vi "GeneratorCpkReport.vi"(4 "结束行in":string, 6 "起始行in":string, 8 "error in (no error)":errorcluster caption="错误输入（无错误）", 10 "测试数据in":string[][](array[string]), 11 "路径in":path) -> (0 "error out":errorcluster caption="错误输出")   [LabVIEW 2020]
uses:
  <vilib>/Utility/NIReport.llb/Report Type.ctl
  <vilib>/addons/_office/_exclsub.llb/font.ctl
  <vilib>/Utility/NIReport.llb/Append Text Table to Report (wrap).vi
  <vilib>/Utility/NIReport.llb/NI_report.lvclass
  <vilib>/Utility/NIReport.llb/NI_ReportGenerationCore.lvlib
  <vilib>/addons/_office/NI_ReportGenerationToolkit.lvlib
  <vilib>/Utility/NIReport.llb/Excel/NI_Excel.lvclass
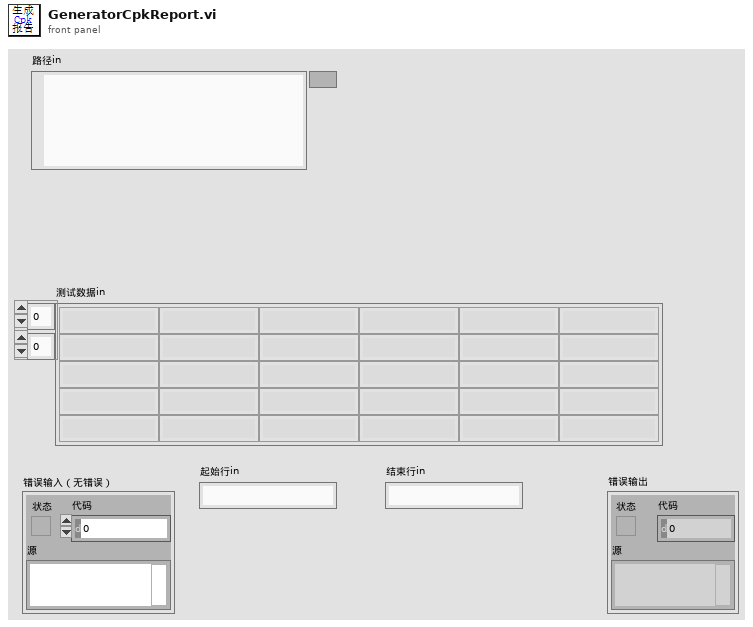
[diagram p1: front panel]
types:
  T1 = cluster{"on/off":bool, "weight":i32, "color":u32}
  T2 = cluster{"position (excel)":cluster{"row":i32, "column":i32}, "name (excel)":string, "bookmark (word)":string}
  T3 = typedef "NI_ReportGenerationToolkit.lvlib/font.ctl" = cluster{"font name":string, "font size":dbl, "bold":u16, "italic":u16, "underline":u16, "strike through":u16, "font color":u32}
  T4 = enum16{"maximized", "minimized", "normal", "no change"}
  T5 = typedef "NI_ReportGenerationCore.lvlib/Report Type.ctl" = enum16{"HTML", "Word", "Excel"}
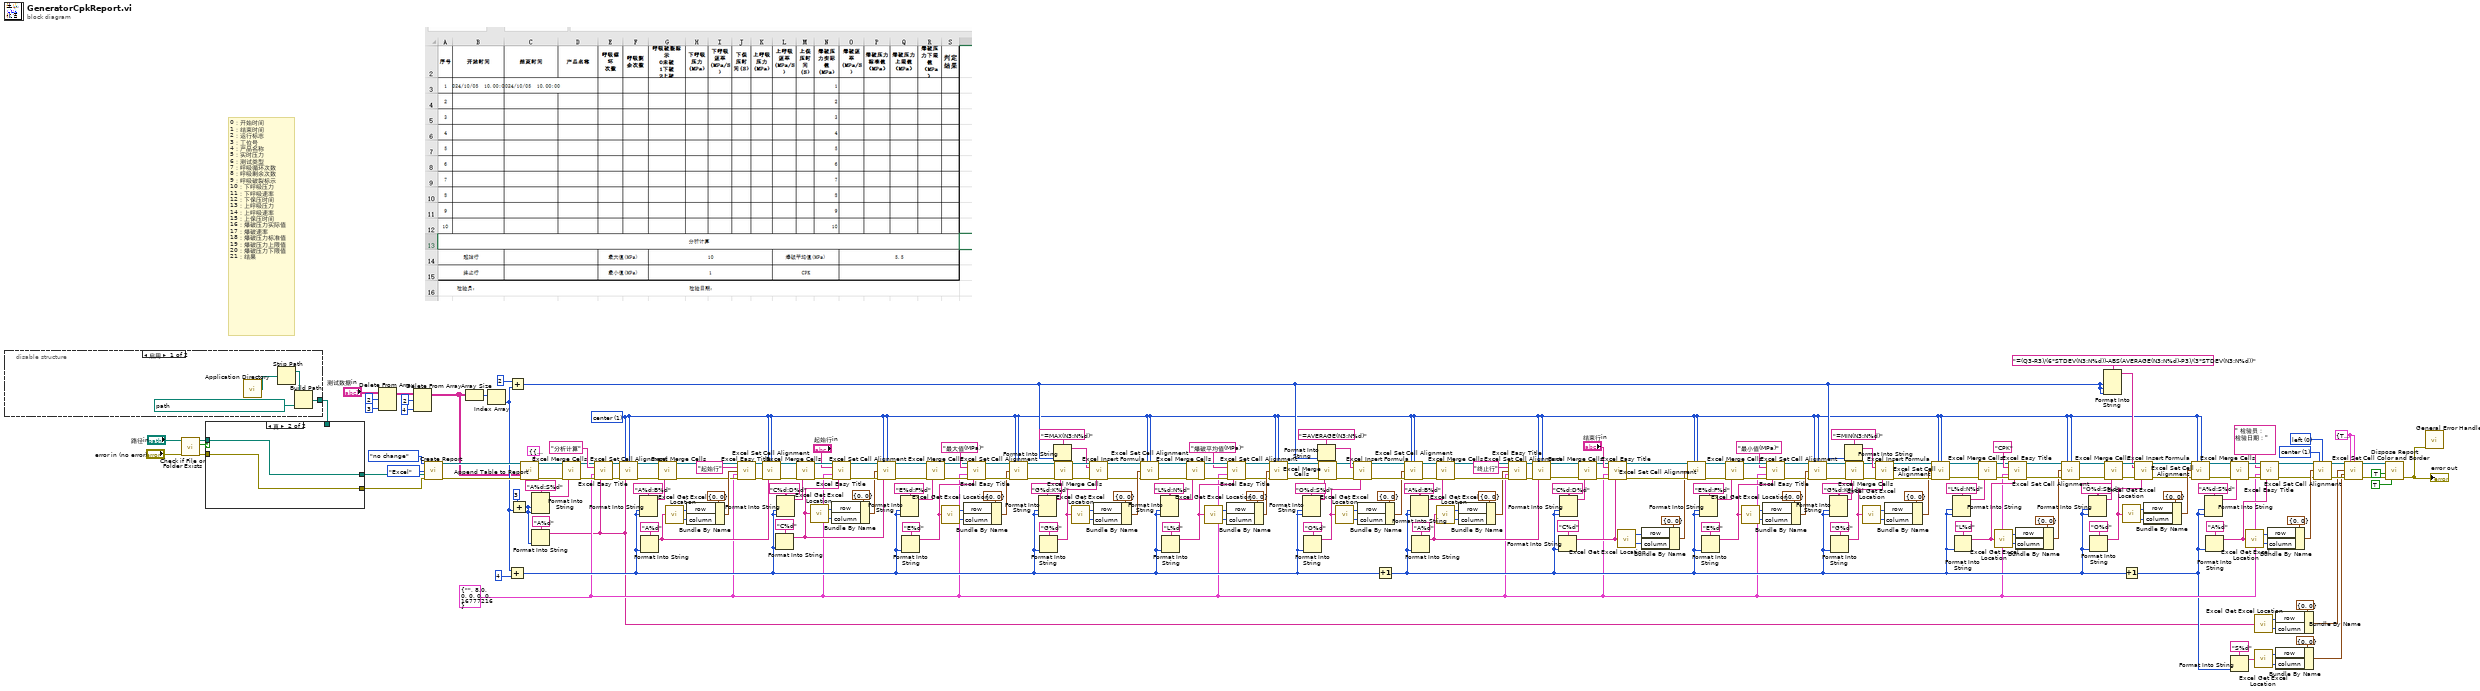
[diagram p0: block diagram]
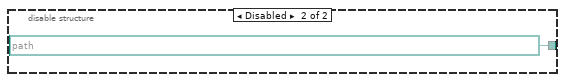
[diagram p2: hidden frame]
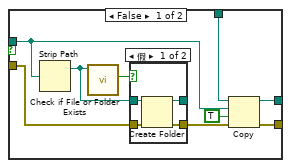
[diagram p3: hidden frame]
diagram:
  w13 = T1 {"on/off"=TRUE, "weight"=2, "color"=0} ("inside border")
  w27 = 0 items=["left", "center", "right"] ("horizontal alignment (left)")
  w28 = 1 items=["top", "center", "bottom"] ("vertical alignment (top)")
  w29 = 1 items=["top", "center", "bottom"] ("vertical alignment (top)")
  w25 = T3 {"font name"="", "font size"=8.0, "bold"=0, "italic"=0, "underline"=0, "strike through"=0, "font color"=16777216} ("font")
  # "0：开始时间\n1：结束时间\n2：运行标志\n3：工位号\n4：产品名称\n5：实时压力\n6：测试类型\n7：呼吸循环次数\n8：呼吸剩余次数\n9：呼吸破裂标示\n10：下呼吸压力\n11：下呼吸速率\n12：下保压时间\n13：上呼吸压力\n14：上呼吸速率\n15：上保压时间\n16：爆破压力实际值\n17：爆破速率\n18：爆破压力标准值\n19：爆破压力上限值\n20：爆破压力下限值\n21：结果"
  n1 = disable-structure shown="启用" {
    disable-tunnel: [w265 path "D:/KebodaWork/深圳何军生/呼吸测试台/SourceCode/Config/呼吸爆破测试CPK最新模板.xlsx" ("appended path")] -> w259
    frame Enabled {
      n2 = call <vilib>:"Application Directory.vi"() -> ("Application Directory"=w264:path)
      n3 = Strip Path(path=w264) -> (stripped path=w263:path)  [unwired: 1 out]
      n4 = Build Path(base path=w263, name or relative path=path "Config/呼吸爆破测试CPK最新模板.xlsx" ("名称或相对路径")) -> (appended path=w265:path)
    }
    frame Disabled {
    }
  }
  n5 = call <vilib>:"Check if File or Folder Exists.vi"("error in (no error)"="error in (no error)", "path"="路径in") -> ("error out"=w261:errorcluster, "file or folder exists?"=w262:bool, "dup path"=w260:path)  [unwired: 7 in]
  n6 = case shown="真" w262 {
    tunnel: w261 -> [w276 w284]
    tunnel: w260 -> [w268 w283]
    tunnel: [w273 w284] -> w253
    tunnel: w259 -> [w270 _]
    tunnel: [w271 w283] -> w254
    frame False {
      n7 = Strip Path(path=w268) -> (stripped path=w275:path)  [unwired: 1 out]
      n8 = call <vilib>:"Check if File or Folder Exists.vi"("path"=w275) -> ("file or folder exists?"=w274:bool)  [unwired: 8 in, 2 out]
      n9 = case shown="假" w274 {
        tunnel: w276 -> [w280 w282]
        tunnel: [w279 w282] -> w269
        tunnel: w275 -> [w278 w281]
        tunnel: [w277 w281] -> _
        frame False {
          n10 = Create Folder(path (use dialog)=w278, error in=w280) -> (created path=w277:path, error out=w279:errorcluster)  [unwired: 1 in, 1 out]
        }
        frame True {
        }
      }
      n11 = Copy(8:w269, 9:TRUE ("覆盖(F)"), 10:w268, 11:w270) -> (0:w273:errorcluster, 3:w271:path)  [unwired: 1 in, 1 out]
    }
    frame True {
    }
  }
  n12 = Delete From Array(array="测试数据in", length=2 ("禁用的索引 (列)"), index (col)=3 ("禁用的索引 (列)")) -> (array with subset deleted=w23:string[][])  [unwired: 1 in, 1 out]
  n13 = Delete From Array(array=w23, length=2 ("禁用的索引 (列)"), index (col)=4 ("禁用的索引 (列)")) -> (array with subset deleted=w20:string[][])  [unwired: 1 in, 1 out]
  n14 = call <vilib>:"Create Report.vi"("window state (normal)"=T4."no change", "report type"=Report_Type."Excel", "template (empty)"=w254, "error in (no error)"=w253) -> ("report out"=w241:refnum<class "NI_report.lvclass">, "error out"=w240:errorcluster)  [unwired: 10 in]
  n15 = Array Size(array=w20) -> (size(s)=w236:i32[])
  n16 = Index Array(array=w236) -> (element=w170:i32)  [unwired: 1 in]
  n17 = Add(x=w170, y=4) -> (x+y=w26:i32)
  n18 = Add(x=2, y=w170) -> (x+y=w46:i32)
  n19 = Add(x=3 ("y"), y=w170) -> (x+y=w226:i32)
  n20 = call-poly <vilib>:"Append Table to Report.vi"("report in"=w241, "MS Office parameters"=T2 {"position (excel)"={"row"=2, "column"=0}, "name (excel)"="", "bookmark (word)"=""}, "text data"=w20, "error in (no error)"=w240) -> ("report out"=w231:refnum<class "NI_report.lvclass">, "error out"=w233:errorcluster)  [unwired: 8 in, 2 out]
  n21 = Format Into String(format string="A%d:S%d" ("格式字符串"), w226, w226) -> (resulting string=w228:string)  [unwired: 2 in, 1 out]
  n22 = Format Into String(format string="A%d" ("格式字符串"), w226) -> (resulting string=w1:string)  [unwired: 2 in, 1 out]
  n23 = call <vilib>:"Excel Merge Cells.vi"("report in"=w231, "error in (no error)"=w233, "name (\"\")"=w228) -> ("report out"=w230:refnum<class "NI_report.lvclass">, "error out"=w232:errorcluster)  [unwired: 11 in]
  n24 = call <vilib>:"Excel Easy Title.vi"("report in"=w230, "title"="分析计算", "font"=w25, "error in (no error)"=w232, "name (\"\")"=w1) -> ("report out"=w225:refnum<class "NI_report.lvclass">, "error out"=w224:errorcluster)  [unwired: 8 in, 1 out]
  n25 = call <vilib>:"Excel Set Cell Alignment.vi"("report in"=w225, "vertical alignment (top)"=w29, "horizontal alignment (left)"=w29, "error in (no error)"=w224, "name (\"\")"=w1) -> ("report out"=w221:refnum<class "NI_report.lvclass">, "error out"=w219:errorcluster)  [unwired: 9 in]
  n26 = Format Into String(format string="A%d:B%d" ("格式字符串"), w26, w26) -> (resulting string=w223:string)  [unwired: 2 in, 1 out]
  n27 = Format Into String(format string="A%d" ("格式字符串"), w26) -> (resulting string=w200:string)  [unwired: 2 in, 1 out]
  n28 = call <vilib>:"Excel Merge Cells.vi"("report in"=w221, "error in (no error)"=w219, "name (\"\")"=w223) -> ("report out"=w220:refnum<class "NI_report.lvclass">, "error out"=w218:errorcluster)  [unwired: 11 in]
  n29 = call <vilib>:"Excel Get Excel Location.vi"("cell's name"=w200) -> ("row"=w248:i32, "column"=w247:i32)
  n30 = Bundle By Name(cluster=cluster{"row":i32, "column":i32} {"row"=0, "column"=0} ("start (0, 0)"), "row"=w248, "column"=w247) -> (w246:cluster{"row":i32, "column":i32})
  n31 = call <vilib>:"Excel Easy Title.vi"("report in"=w220, "title"="起始行", "start (0, 0)"=w246, "font"=w25, "error in (no error)"=w218) -> ("report out"=w214:refnum<class "NI_report.lvclass">, "error out"=w215:errorcluster)  [unwired: 8 in, 1 out]
  n32 = call <vilib>:"Excel Set Cell Alignment.vi"("report in"=w214, "vertical alignment (top)"=w29, "horizontal alignment (left)"=w29, "error in (no error)"=w215, "name (\"\")"=w200) -> ("report out"=w201:refnum<class "NI_report.lvclass">, "error out"=w202:errorcluster)  [unwired: 9 in]
  n33 = Format Into String(format string="C%d" ("格式字符串"), w26) -> (resulting string=w165:string)  [unwired: 2 in, 1 out]
  n34 = Format Into String(format string="C%d:D%d" ("格式字符串"), w26, w26) -> (resulting string=w208:string)  [unwired: 2 in, 1 out]
  n35 = call <vilib>:"Excel Merge Cells.vi"("report in"=w201, "error in (no error)"=w202, "name (\"\")"=w208) -> ("report out"=w210:refnum<class "NI_report.lvclass">, "error out"=w211:errorcluster)  [unwired: 11 in]
  n36 = call <vilib>:"Excel Get Excel Location.vi"("cell's name"=w165) -> ("row"=w205:i32, "column"=w206:i32)
  n37 = Bundle By Name(cluster=cluster{"row":i32, "column":i32} {"row"=0, "column"=0} ("start (0, 0)"), "row"=w205, "column"=w206) -> (w166:cluster{"row":i32, "column":i32})
  n38 = call <vilib>:"Excel Easy Title.vi"("report in"=w210, "title"="起始行in", "font"=w25, "error in (no error)"=w211, "name (\"\")"=w165) -> ("report out"=w213:refnum<class "NI_report.lvclass">, "error out"=w212:errorcluster)  [unwired: 8 in, 1 out]
  n39 = call <vilib>:"Excel Set Cell Alignment.vi"("report in"=w213, "vertical alignment (top)"=w29, "horizontal alignment (left)"=w29, "start (-1, -1)"=w166, "error in (no error)"=w212, "name (\"\")"=w165) -> ("report out"=w187:refnum<class "NI_report.lvclass">, "error out"=w188:errorcluster)  [unwired: 8 in]
  n40 = Format Into String(format string="E%d:F%d" ("格式字符串"), w26, w26) -> (resulting string=w194:string)  [unwired: 2 in, 1 out]
  n41 = Format Into String(format string="E%d" ("格式字符串"), w26) -> (resulting string=w167:string)  [unwired: 2 in, 1 out]
  n42 = call <vilib>:"Excel Merge Cells.vi"("report in"=w187, "error in (no error)"=w188, "name (\"\")"=w194) -> ("report out"=w195:refnum<class "NI_report.lvclass">, "error out"=w196:errorcluster)  [unwired: 11 in]
  n43 = call <vilib>:"Excel Get Excel Location.vi"("cell's name"=w167) -> ("row"=w192:i32, "column"=w193:i32)
  n44 = Bundle By Name(cluster=cluster{"row":i32, "column":i32} {"row"=0, "column"=0} ("start (0, 0)"), "row"=w192, "column"=w193) -> (w168:cluster{"row":i32, "column":i32})
  n45 = call <vilib>:"Excel Easy Title.vi"("report in"=w195, "title"="最大值(MPa)", "font"=w25, "error in (no error)"=w196, "name (\"\")"=w167) -> ("report out"=w199:refnum<class "NI_report.lvclass">, "error out"=w198:errorcluster)  [unwired: 8 in, 1 out]
  n46 = call <vilib>:"Excel Set Cell Alignment.vi"("report in"=w199, "vertical alignment (top)"=w29, "horizontal alignment (left)"=w29, "start (-1, -1)"=w168, "error in (no error)"=w198) -> ("report out"=w171:refnum<class "NI_report.lvclass">, "error out"=w172:errorcluster)  [unwired: 9 in]
  n47 = Format Into String(format string="G%d:K%d" ("格式字符串"), w26, w26) -> (resulting string=w181:string)  [unwired: 2 in, 1 out]
  n48 = Format Into String(format string="G%d" ("格式字符串"), w26) -> (resulting string=w178:string)  [unwired: 2 in, 1 out]
  n49 = Format Into String(format string="=MAX(N3:N%d)" ("格式字符串"), w46) -> (resulting string=w173:string)  [unwired: 2 in, 1 out]
  n50 = call <vilib>:"Excel Merge Cells.vi"("report in"=w171, "error in (no error)"=w172, "name (\"\")"=w181) -> ("report out"=w175:refnum<class "NI_report.lvclass">, "error out"=w177:errorcluster)  [unwired: 11 in]
  n51 = call <vilib>:"Excel Get Excel Location.vi"("cell's name"=w178) -> ("row"=w183:i32, "column"=w182:i32)
  n52 = call <vilib>:"Excel Insert Formula.vi"("report in"=w175, "formula"=w173, "error in (no error)"=w177, "name (\"\")"=w178) -> ("report out"=w174:refnum<class "NI_report.lvclass">, "error out"=w176:errorcluster)  [unwired: 10 in]
  n53 = Bundle By Name(cluster=cluster{"row":i32, "column":i32} {"row"=0, "column"=0} ("start (0, 0)"), "row"=w183, "column"=w182) -> (w179:cluster{"row":i32, "column":i32})
  n54 = call <vilib>:"Excel Set Cell Alignment.vi"("report in"=w174, "vertical alignment (top)"=w29, "horizontal alignment (left)"=w29, "start (-1, -1)"=w179, "error in (no error)"=w176) -> ("report out"=w150:refnum<class "NI_report.lvclass">, "error out"=w151:errorcluster)  [unwired: 9 in]
  n55 = Format Into String(format string="L%d:N%d" ("格式字符串"), w26, w26) -> (resulting string=w157:string)  [unwired: 2 in, 1 out]
  n56 = Format Into String(format string="L%d" ("格式字符串"), w26) -> (resulting string=w164:string)  [unwired: 2 in, 1 out]
  n57 = call <vilib>:"Excel Merge Cells.vi"("report in"=w150, "error in (no error)"=w151, "name (\"\")"=w157) -> ("report out"=w156:refnum<class "NI_report.lvclass">, "error out"=w155:errorcluster)  [unwired: 11 in]
  n58 = call <vilib>:"Excel Get Excel Location.vi"("cell's name"=w164) -> ("row"=w159:i32, "column"=w158:i32)
  n59 = Bundle By Name(cluster=cluster{"row":i32, "column":i32} {"row"=0, "column"=0} ("start (0, 0)"), "row"=w159, "column"=w158) -> (w163:cluster{"row":i32, "column":i32})
  n60 = call <vilib>:"Excel Easy Title.vi"("report in"=w156, "title"="爆破平均值(MPa)", "font"=w25, "error in (no error)"=w155, "name (\"\")"=w164) -> ("report out"=w152:refnum<class "NI_report.lvclass">, "error out"=w153:errorcluster)  [unwired: 8 in, 1 out]
  n61 = call <vilib>:"Excel Set Cell Alignment.vi"("report in"=w152, "vertical alignment (top)"=w29, "horizontal alignment (left)"=w29, "start (-1, -1)"=w163, "error in (no error)"=w153) -> ("report out"=w134:refnum<class "NI_report.lvclass">, "error out"=w135:errorcluster)  [unwired: 9 in]
  n62 = Format Into String(format string="O%d:S%d" ("格式字符串"), w26, w26) -> (resulting string=w141:string)  [unwired: 2 in, 1 out]
  n63 = Format Into String(format string="O%d" ("格式字符串"), w26) -> (resulting string=w144:string)  [unwired: 2 in, 1 out]
  n64 = Format Into String(format string="=AVERAGE(N3:N%d)" ("格式字符串"), w46) -> (resulting string=w149:string)  [unwired: 2 in, 1 out]
  n65 = call <vilib>:"Excel Merge Cells.vi"("report in"=w134, "error in (no error)"=w135, "name (\"\")"=w141) -> ("report out"=w147:refnum<class "NI_report.lvclass">, "error out"=w145:errorcluster)  [unwired: 11 in]
  n66 = call <vilib>:"Excel Get Excel Location.vi"("cell's name"=w144) -> ("row"=w139:i32, "column"=w140:i32)
  n67 = call <vilib>:"Excel Insert Formula.vi"("report in"=w147, "formula"=w149, "error in (no error)"=w145, "name (\"\")"=w144) -> ("report out"=w148:refnum<class "NI_report.lvclass">, "error out"=w146:errorcluster)  [unwired: 10 in]
  n68 = Bundle By Name(cluster=cluster{"row":i32, "column":i32} {"row"=0, "column"=0} ("start (0, 0)"), "row"=w139, "column"=w140) -> (w143:cluster{"row":i32, "column":i32})
  n69 = Increment(x=w26) -> (x+1=w30:i32)
  n70 = call <vilib>:"Excel Set Cell Alignment.vi"("report in"=w148, "vertical alignment (top)"=w29, "horizontal alignment (left)"=w29, "start (-1, -1)"=w143, "error in (no error)"=w146) -> ("report out"=w119:refnum<class "NI_report.lvclass">, "error out"=w120:errorcluster)  [unwired: 9 in]
  n71 = Format Into String(format string="A%d:B%d" ("格式字符串"), w30, w30) -> (resulting string=w126:string)  [unwired: 2 in, 1 out]
  n72 = Format Into String(format string="A%d" ("格式字符串"), w30) -> (resulting string=w133:string)  [unwired: 2 in, 1 out]
  n73 = call <vilib>:"Excel Merge Cells.vi"("report in"=w119, "error in (no error)"=w120, "name (\"\")"=w126) -> ("report out"=w128:refnum<class "NI_report.lvclass">, "error out"=w129:errorcluster)  [unwired: 11 in]
  n74 = call <vilib>:"Excel Get Excel Location.vi"("cell's name"=w133) -> ("row"=w122:i32, "column"=w123:i32)
  n75 = Bundle By Name(cluster=cluster{"row":i32, "column":i32} {"row"=0, "column"=0} ("start (0, 0)"), "row"=w122, "column"=w123) -> (w124:cluster{"row":i32, "column":i32})
  n76 = call <vilib>:"Excel Easy Title.vi"("report in"=w128, "title"="终止行", "start (0, 0)"=w124, "font"=w25, "error in (no error)"=w129) -> ("report out"=w132:refnum<class "NI_report.lvclass">, "error out"=w131:errorcluster)  [unwired: 8 in, 1 out]
  n77 = call <vilib>:"Excel Set Cell Alignment.vi"("report in"=w132, "vertical alignment (top)"=w29, "horizontal alignment (left)"=w29, "error in (no error)"=w131, "name (\"\")"=w133) -> ("report out"=w114:refnum<class "NI_report.lvclass">, "error out"=w113:errorcluster)  [unwired: 9 in]
  n78 = Format Into String(format string="C%d" ("格式字符串"), w30) -> (resulting string=w109:string)  [unwired: 2 in, 1 out]
  n79 = Format Into String(format string="C%d:D%d" ("格式字符串"), w30, w30) -> (resulting string=w118:string)  [unwired: 2 in, 1 out]
  n80 = call <vilib>:"Excel Merge Cells.vi"("report in"=w114, "error in (no error)"=w113, "name (\"\")"=w118) -> ("report out"=w116:refnum<class "NI_report.lvclass">, "error out"=w115:errorcluster)  [unwired: 11 in]
  n81 = call <vilib>:"Excel Easy Title.vi"("report in"=w116, "title"="结束行in", "font"=w25, "error in (no error)"=w115, "name (\"\")"=w109) -> ("report out"=w111:refnum<class "NI_report.lvclass">, "error out"=w112:errorcluster)  [unwired: 8 in, 1 out]
  n82 = call <vilib>:"Excel Get Excel Location.vi"("cell's name"=w109) -> ("row"=w244:i32, "column"=w245:i32)
  n83 = Bundle By Name(cluster=cluster{"row":i32, "column":i32} {"row"=0, "column"=0} ("start (0, 0)"), "row"=w244, "column"=w245) -> (w110:cluster{"row":i32, "column":i32})
  n84 = call <vilib>:"Excel Set Cell Alignment.vi"("report in"=w111, "vertical alignment (top)"=w29, "horizontal alignment (left)"=w29, "start (-1, -1)"=w110, "error in (no error)"=w112) -> ("report out"=w95:refnum<class "NI_report.lvclass">, "error out"=w94:errorcluster)  [unwired: 9 in]
  n85 = Format Into String(format string="E%d:F%d" ("格式字符串"), w30, w30) -> (resulting string=w101:string)  [unwired: 2 in, 1 out]
  n86 = Format Into String(format string="E%d" ("格式字符串"), w30) -> (resulting string=w108:string)  [unwired: 2 in, 1 out]
  n87 = call <vilib>:"Excel Merge Cells.vi"("report in"=w95, "error in (no error)"=w94, "name (\"\")"=w101) -> ("report out"=w100:refnum<class "NI_report.lvclass">, "error out"=w99:errorcluster)  [unwired: 11 in]
  n88 = call <vilib>:"Excel Get Excel Location.vi"("cell's name"=w108) -> ("row"=w103:i32, "column"=w102:i32)
  n89 = Bundle By Name(cluster=cluster{"row":i32, "column":i32} {"row"=0, "column"=0} ("start (0, 0)"), "row"=w103, "column"=w102) -> (w107:cluster{"row":i32, "column":i32})
  n90 = call <vilib>:"Excel Easy Title.vi"("report in"=w100, "title"="最小值(MPa)", "font"=w25, "error in (no error)"=w99, "name (\"\")"=w108) -> ("report out"=w96:refnum<class "NI_report.lvclass">, "error out"=w97:errorcluster)  [unwired: 8 in, 1 out]
  n91 = call <vilib>:"Excel Set Cell Alignment.vi"("report in"=w96, "vertical alignment (top)"=w29, "horizontal alignment (left)"=w29, "start (-1, -1)"=w107, "error in (no error)"=w97) -> ("report out"=w79:refnum<class "NI_report.lvclass">, "error out"=w78:errorcluster)  [unwired: 9 in]
  n92 = Format Into String(format string="G%d:K%d" ("格式字符串"), w30, w30) -> (resulting string=w85:string)  [unwired: 2 in, 1 out]
  n93 = Format Into String(format string="G%d" ("格式字符串"), w30) -> (resulting string=w88:string)  [unwired: 2 in, 1 out]
  n94 = Format Into String(format string="=MIN(N3:N%d)" ("格式字符串"), w46) -> (resulting string=w93:string)  [unwired: 2 in, 1 out]
  n95 = call <vilib>:"Excel Merge Cells.vi"("report in"=w79, "error in (no error)"=w78, "name (\"\")"=w85) -> ("report out"=w91:refnum<class "NI_report.lvclass">, "error out"=w89:errorcluster)  [unwired: 11 in]
  n96 = call <vilib>:"Excel Get Excel Location.vi"("cell's name"=w88) -> ("row"=w83:i32, "column"=w84:i32)
  n97 = call <vilib>:"Excel Insert Formula.vi"("report in"=w91, "formula"=w93, "error in (no error)"=w89, "name (\"\")"=w88) -> ("report out"=w92:refnum<class "NI_report.lvclass">, "error out"=w90:errorcluster)  [unwired: 10 in]
  n98 = Bundle By Name(cluster=cluster{"row":i32, "column":i32} {"row"=0, "column"=0} ("start (0, 0)"), "row"=w83, "column"=w84) -> (w87:cluster{"row":i32, "column":i32})
  n99 = call <vilib>:"Excel Set Cell Alignment.vi"("report in"=w92, "vertical alignment (top)"=w29, "horizontal alignment (left)"=w29, "start (-1, -1)"=w87, "error in (no error)"=w90) -> ("report out"=w64:refnum<class "NI_report.lvclass">, "error out"=w63:errorcluster)  [unwired: 9 in]
  n100 = Format Into String(format string="L%d:N%d" ("格式字符串"), w30, w30) -> (resulting string=w72:string)  [unwired: 2 in, 1 out]
  n101 = Format Into String(format string="L%d" ("格式字符串"), w30) -> (resulting string=w65:string)  [unwired: 2 in, 1 out]
  n102 = call <vilib>:"Excel Merge Cells.vi"("report in"=w64, "error in (no error)"=w63, "name (\"\")"=w72) -> ("report out"=w73:refnum<class "NI_report.lvclass">, "error out"=w74:errorcluster)  [unwired: 11 in]
  n103 = call <vilib>:"Excel Get Excel Location.vi"("cell's name"=w65) -> ("row"=w70:i32, "column"=w71:i32)
  n104 = call <vilib>:"Excel Easy Title.vi"("report in"=w73, "title"="CPK", "font"=w25, "error in (no error)"=w74, "name (\"\")"=w65) -> ("report out"=w77:refnum<class "NI_report.lvclass">, "error out"=w76:errorcluster)  [unwired: 8 in, 1 out]
  n105 = Bundle By Name(cluster=cluster{"row":i32, "column":i32} {"row"=0, "column"=0} ("start (0, 0)"), "row"=w70, "column"=w71) -> (w66:cluster{"row":i32, "column":i32})
  n106 = call <vilib>:"Excel Set Cell Alignment.vi"("report in"=w77, "vertical alignment (top)"=w29, "horizontal alignment (left)"=w29, "start (-1, -1)"=w66, "error in (no error)"=w76) -> ("report out"=w48:refnum<class "NI_report.lvclass">, "error out"=w47:errorcluster)  [unwired: 9 in]
  n107 = Format Into String(format string="O%d:S%d" ("格式字符串"), w30, w30) -> (resulting string=w57:string)  [unwired: 2 in, 1 out]
  n108 = Format Into String(format string="O%d" ("格式字符串"), w30) -> (resulting string=w54:string)  [unwired: 2 in, 1 out]
  n109 = Format Into String(format string="=(Q3-R3)/(6*STDEV(N3:N%d))-ABS(AVERAGE(N3:N%d)-P3)/(3*STDEV(N3:N%d))" ("格式字符串"), w46, w46, w46) -> (resulting string=w49:string)  [unwired: 2 in, 1 out]
  n110 = call <vilib>:"Excel Merge Cells.vi"("report in"=w48, "error in (no error)"=w47, "name (\"\")"=w57) -> ("report out"=w51:refnum<class "NI_report.lvclass">, "error out"=w53:errorcluster)  [unwired: 11 in]
  n111 = call <vilib>:"Excel Get Excel Location.vi"("cell's name"=w54) -> ("row"=w59:i32, "column"=w58:i32)
  n112 = Increment(x=w30) -> (x+1=w2:i32)
  n113 = call <vilib>:"Excel Insert Formula.vi"("report in"=w51, "formula"=w49, "error in (no error)"=w53, "name (\"\")"=w54) -> ("report out"=w50:refnum<class "NI_report.lvclass">, "error out"=w52:errorcluster)  [unwired: 10 in]
  n114 = Bundle By Name(cluster=cluster{"row":i32, "column":i32} {"row"=0, "column"=0} ("start (0, 0)"), "row"=w59, "column"=w58) -> (w55:cluster{"row":i32, "column":i32})
  n115 = call <vilib>:"Excel Set Cell Alignment.vi"("report in"=w50, "vertical alignment (top)"=w29, "horizontal alignment (left)"=w29, "start (-1, -1)"=w55, "error in (no error)"=w52) -> ("report out"=w31:refnum<class "NI_report.lvclass">, "error out"=w32:errorcluster)  [unwired: 9 in]
  n116 = Format Into String(format string="A%d:S%d" ("格式字符串"), w2, w2) -> (resulting string=w38:string)  [unwired: 2 in, 1 out]
  n117 = Format Into String(format string="A%d" ("格式字符串"), w2) -> (resulting string=w45:string)  [unwired: 2 in, 1 out]
  n118 = call <vilib>:"Excel Merge Cells.vi"("report in"=w31, "error in (no error)"=w32, "name (\"\")"=w38) -> ("report out"=w37:refnum<class "NI_report.lvclass">, "error out"=w36:errorcluster)  [unwired: 11 in]
  n119 = Format Into String(format string="S%d" ("格式字符串"), w2) -> (resulting string=w3:string)  [unwired: 2 in, 1 out]
  n120 = call <vilib>:"Excel Get Excel Location.vi"("cell's name"=w45) -> ("row"=w40:i32, "column"=w39:i32)
  n121 = call <vilib>:"Excel Get Excel Location.vi"("cell's name"=w1) -> ("row"=w11:i32, "column"=w12:i32)
  n122 = call <vilib>:"Excel Get Excel Location.vi"("cell's name"=w3) -> ("row"=w8:i32, "column"=w9:i32)
  n123 = call <vilib>:"Excel Easy Title.vi"("report in"=w37, "title"=" 检验员：                                                                         检验日期：", "font"=w25, "error in (no error)"=w36, "name (\"\")"=w45) -> ("report out"=w33:refnum<class "NI_report.lvclass">, "error out"=w34:errorcluster)  [unwired: 8 in, 1 out]
  n124 = Bundle By Name(cluster=cluster{"row":i32, "column":i32} {"row"=0, "column"=0} ("start (0, 0)"), "row"=w40, "column"=w39) -> (w44:cluster{"row":i32, "column":i32})
  n125 = Bundle By Name(cluster=cluster{"row":i32, "column":i32} {"row"=0, "column"=0} ("start (0, 0)"), "row"=w11, "column"=w12) -> (w6:cluster{"row":i32, "column":i32})
  n126 = Bundle By Name(cluster=cluster{"row":i32, "column":i32} {"row"=0, "column"=0} ("start (0, 0)"), "row"=w8, "column"=w9) -> (w5:cluster{"row":i32, "column":i32})
  n127 = call <vilib>:"Excel Set Cell Alignment.vi"("report in"=w33, "vertical alignment (top)"=w28, "horizontal alignment (left)"=w27, "start (-1, -1)"=w44, "error in (no error)"=w34) -> ("report out"=w17:refnum<class "NI_report.lvclass">, "error out"=w16:errorcluster)  [unwired: 9 in]
  n128 = call <vilib>:"Excel Set Cell Color and Border.vi"("report in"=w17, "inside border"=w13, "outside border"=w13, "start (-1, -1)"=w6, "end (-1, -1)"=w5, "error in (no error)"=w16) -> ("report out"=w15:refnum<class "NI_report.lvclass">, "error out"=w14:errorcluster)  [unwired: 8 in]
  n129 = call-dynamic "Dispose Report.vi"("report in"=w15, "save changes? (F)"=TRUE, "error in (no error)"=w14, "close report? (T)"=TRUE) -> ("error out"=w250:errorcluster)  [unwired: 11 in]
  "error out" <- w250
  n130 = call <vilib>:"General Error Handler.vi"("error in (no error)"=w250) -> ()  [unwired: 10 in, 5 out]
